vi "Craigslist Textbooks for Fusion Table V3.vi"() -> ()   [LabVIEW 2010]
uses:
  <vilib>/Utility/file.llb/Read From Spreadsheet File (string).vi
  <vilib>/Utility/file.llb/Write To Spreadsheet File (string).vi
panel:
  out "File Save Path":string
  out "Array":string[][](array[string])
  out "user books per city":string[][](array[string])
  out "Final filtered":string[][](array[string])
  out "element":string
  out "All closest city data":string[](array[string])
  out "All Data":string[][](array[string])
  out "ID number":string
  in  "Geo Locations 2":string[][](array[string])=[["http://boulder.craigslist.org/bks/", "http://boulder.craigslist.org/bks/index100.html", "http://boulder.craigslist.org/bks/index200.html", "http://boulder.craigslist.org/bks/index300.html", "http://boulder.craigslist.org/bks/index400.html", "http://boulder.craigslist.org/bks/index500.html", "http://boulder.craigslist.org/bks/index600.html", "http://boulder.craigslist.org/bks/index700.html", "http://boulder.craigslist.org/bks/index800.html", "http://boulder.craigslist.org/bks/index900.html", "40.006846", "-105.271575", "CU Boulder", "Boulder", "CO", "4/30/2004 7:48:47 PM", "3558694"], ["http://phoenix.craigslist.org/bks/", "http://phoenix.craigslist.org/bks/index100.html", "http://phoenix.craigslist.org/bks/index200.html", "http://phoenix.craigslist.org/bks/index300.html", "http://phoenix.craigslist.org/bks/index400.html", "http://phoenix.craigslist.org/bks/index500.html", "http://phoenix.craigslist.org/bks/index600.html", "http://phoenix.craigslist.org/bks/index700.html", "http://phoenix.craigslist.org/bks/index800.html", "http://phoenix.craigslist.org/bks/index900.html", "33.416147", "-111.938152", "ASU Arizona State University", "Phoenix", "AZ", "4/30/2004 7:48:47 PM", "3558688"], ["http://orlando.craigslist.org/bks/", "http://orlando.craigslist.org/bks/index100.html", "http://orlando.craigslist.org/bks/index200.html", "http://orlando.craigslist.org/bks/index300.html", "http://orlando.craigslist.org/bks/index400.html", "http://orlando.craigslist.org/bks/index500.html", "http://orlando.craigslist.org/bks/index600.html", "http://orlando.craigslist.org/bks/index700.html", "http://orlando.craigslist.org/bks/index800.html", "http://orlando.craigslist.org/bks/index900.html", "28.602326", "-81.19994", "UCF University of Central Florida", "orlando", "FL", "", "3558796"], ["http://austin.craigslist.org/bks/", "http://austin.craigslist.org/bks/index100.html", "http://austin.craigslist.org/bks/index200.html", "http://austin.craigslist.org/bks/index300.html", "http://austin.craigslist.org/bks/index400.html", "http://austin.craigslist.org/bks/index500.html", "http://austin.craigslist.org/bks/index600.html", "http://austin.craigslist.org/bks/index700.html", "http://austin.craigslist.org/bks/index800.html", "http://austin.craigslist.org/bks/index900.html", "30.28629", "-97.740211", "UT Austin University of Texas at Austin", "Austin", "TX", "40.006846", "3588692"], ["http://columbus.craigslist.org/bks/", "http://columbus.craigslist.org/bks/index100.html", "http://columbus.craigslist.org/bks/index200.html", "http:/columbus.craigslist.org/bks/index300.html", "http://columbus.craigslist.org/bks/index400.html", "http://columbus.craigslist.org/bks/index500.html", "http://columbus.craigslist.org/bks/index600.html", "http://columbus.craigslist.org/bks/index700.html", "http://columbus.craigslist.org/bks/index800.html", "http://columbus.craigslist.org/bks/index900.html", "40.000778", "-83.010421", "OSU Ohio State University", "Columbus", "OH", "4/30/2004 7:48:47 PM", "3558876"], ["http://minneapolis.craigslist.org/bks/", "http://minneapolis.craigslist.org/bks/index100.html", "http://minneapolis.craigslist.org/bks/index200.html", "http://minneapolis.craigslist.org/bks/index300.html", "http://minneapolis.craigslist.org/bks/index400.html", "http://minneapolis.craigslist.org/bks/index500.html", "http://minneapolis.craigslist.org/bks/index600.html", "http://minneapolis.craigslist.org/bks/index700.html", "http://minneapolis.craigslist.org/bks/index800.html", "http://minneapolis.craigslist.org/bks/index900.html", "44.974999", "-93.231847", "U of M University of Minnesota", "minneapolis", "MN", "", "3558694"], ["http://losangeles.craigslist.org/lac/bks/", "http://losangeles.craigslist.org/lac/bks/index100.html", "http://losangeles.craigslist.org/lac/bks/index200.html", "http://losangeles.craigslist.org/lac/bks/index300.html", "http://losangeles.craigslist.org/lac/bks/index400.html", "http://losangeles.craigslist.org/lac/bks/index500.html", "http://losangeles.craigslist.org/lac/bks/index600.html", "http://losangeles.craigslist.org/lac/bks/index700.html", "http://losangeles.craigslist.org/lac/bks/index800.html", "http://losangeles.craigslist.org/lac/bks/index900.html", "34.020612", "-118.284409", "USC University of Southern California", "USC", "CA", "40.006846", "3588399"], ["http://boston.craigslist.org/gbs/bks/", "http://boston.craigslist.org/gbs/bks/index100.html", "http://boston.craigslist.org/gbs/bks/index200.html", "http://boston.craigslist.org/gbs/bks/index300.html", "http://boston.craigslist.org/gbs/bks/index400.html", "http://boston.craigslist.org/gbs/bks/index500.html", "http://boston.craigslist.org/gbs/bks/index600.html", "http://boston.craigslist.org/gbs/bks/index700.html", "http://boston.craigslist.org/gbs/bks/index800.html", "http://boston.craigslist.org/gbs/bks/index900.html", "42.372852", "-71.117581", "Harvard University", "Cambridge", "MA", "40.006846", "3589108"], ["http://newhaven.craigslist.org/bks/", "http://newhaven.craigslist.org/bks/index100.html", "http://newhaven.craigslist.org/bks/index200.html", "http://newhaven.craigslist.org/bks/index300.html", "http://newhaven.craigslist.org/bks/index400.html", "http://newhaven.craigslist.org/bks/index500.html", "http://newhaven.craigslist.org/bks/index600.html", "http://newhaven.craigslist.org/bks/index700.html", "http://newhaven.craigslist.org/bks/index800.html", "http://newhaven.craigslist.org/bks/index900.html", "41.311211", "-72.928662", "Yale University", "New Haven", "CT", "40.006846", "3588844"], ["http://sfbay.craigslist.org/pen/bks/", "http://sfbay.craigslist.org/pen/bks/index100.html", "http://sfbay.craigslist.org/pen/bks/index200.html", "http://sfbay.craigslist.org/pen/bks/index300.html", "http://sfbay.craigslist.org/pen/bks/index400.html", "http://sfbay.craigslist.org/pen/bks/index500.html", "http://sfbay.craigslist.org/pen/bks/index600.html", "http://sfbay.craigslist.org/pen/bks/index700.html", "http://sfbay.craigslist.org/pen/index800.html", "http://sfbay.craigslist.org/pen/bks/index900.html", "37.425576", "-122.168891", "Stanford University", "Redwood City", "CA", "40.006846", "3588839"], ["http://chicago.craigslist.org/nch/bks/", "http://chicago.craigslist.org/nch/bks/index100.html", "http://chicago.craigslist.org/nch/bks/index200.html", "http://chicago.craigslist.org/nch/bks/index300.html", "http://chicago.craigslist.org/nch/bks/index400.html", "http://chicago.craigslist.org/nch/bks/index500.html", "http://chicago.craigslist.org/nch/bks/index600.html", "http://chicago.craigslist.org/nch/bks/index700.html", "http://chicago.craigslist.org/nch/bks/index800.html", "http://chicago.craigslist.org/nch/bks/index900.html", "42.057801", "-87.67563", "NU Northwestern University", "Evanston", "IL", "40.006846", "3588099"], ["http://sfbay.craigslist.org/eby/bks/", "http://sfbay.craigslist.org/eby/bks/index100.html", "http://sfbay.craigslist.org/eby/bks/index200.html", "http://sfbay.craigslist.org/eby/bks/index300.html", "http://sfbay.craigslist.org/eby/bks/index400.html", "http://sfbay.craigslist.org/eby/bks/index500.html", "http://sfbay.craigslist.org/eby/bks/index600.html", "http://sfbay.craigslist.org/eby/bks/index700.html", "http://sfbay.craigslist.org/eby/bks/index800.html", "http://sfbay.craigslist.org/eby/bks/index900.html", "37.872296", "-122.258799", "UC Berkeley University of California at Berkeley", "Berkeley", "CA", "40.006846", "3588671"], ["http://fortcollins.craigslist.org/bks/", "http://fortcollins.craigslist.org/bks/index100.html", "http://fortcollins.craigslist.org/bks/index200.html", "http://fortcollins.craigslist.org/bks/index300.html", "http://fortcollins.craigslist.org/bks/index400.html", "http://fortcollins.craigslist.org/bks/index500.html", "http://fortcollins.craigslist.org/bks/index600.html", "http://fortcollins.craigslist.org/bks/index700.html", "http://fortcollins.craigslist.org/bks/index800.html", "http://fortcollins.craigslist.org/bks/index900.html", "40.571556", "-105.080624", "CSU Colorado State University", "Fort Collins", "CO", "40.006846", "3589102"], ["http://denver.craigslist.org/bks/", "http://denver.craigslist.org/bks/index100.html", "http://denver.craigslist.org/bks/index200.html", "http://denver.craigslist.org/bks/index300.html", "http://denver.craigslist.org/bks/index400.html", "http://denver.craigslist.org/bks/index500.html", "http://denver.craigslist.org/bks/index600.html", "http://denver.craigslist.org/bks/index700.html", "http://denver.craigslist.org/bks/index800.html", "http://denver.craigslist.org/bks/index900.html", "39.676707", "-104.962628", "DU University of Denver", "Denver", "CO", "40.006846", "3588279"], ["http://boston.craigslist.org/gbs/bks/", "http://boston.craigslist.org/gbs/bks/index100.html", "http://boston.craigslist.org/gbs/bks/index200.html", "http://boston.craigslist.org/gbs/bks/index300.html", "http://boston.craigslist.org/gbs/bks/index400.html", "http://boston.craigslist.org/gbs/bks/index500.html", "http://boston.craigslist.org/gbs/bks/index600.html", "http://boston.craigslist.org/gbs/bks/index700.html", "http://boston.craigslist.org/gbs/bks/index800.html", "http://boston.craigslist.org/gbs/bks/index900.html", "42.361556", "-71.090759", "MIT Massachusetts Institute of Technology", "Cambridge", "MA", "40.006846", "3588278"]]
  out "Finished Array":string[][](array[string])
  out "One Row Edited":string[](array[string])
  out "Craigslist Link":string
  out "Place":string
  out "One Row Unedited":string[](array[string])
  out "Category":string
  out "Extra Information":string
  out "Price":string
  out "General Location":string
  out "Time":string
  out "Date":string
  out "Year":string
  out "Date, Time":string
  out "State":string
  out "City":string
  out "long string":string
  out "lat string":string
  out "Full Source":string
  out "long":dbl
  out "lat":dbl
  out "Body":string
  out "E-mail Contact":string
  out "Title":string
  out "Parse Count":i32
  out "Current Page Source":string
  # "http://thestudentbookproject.org/index2.php?option=com_google_maps_boulder&task=dynamic&no_html=1&download=true&zip=false"
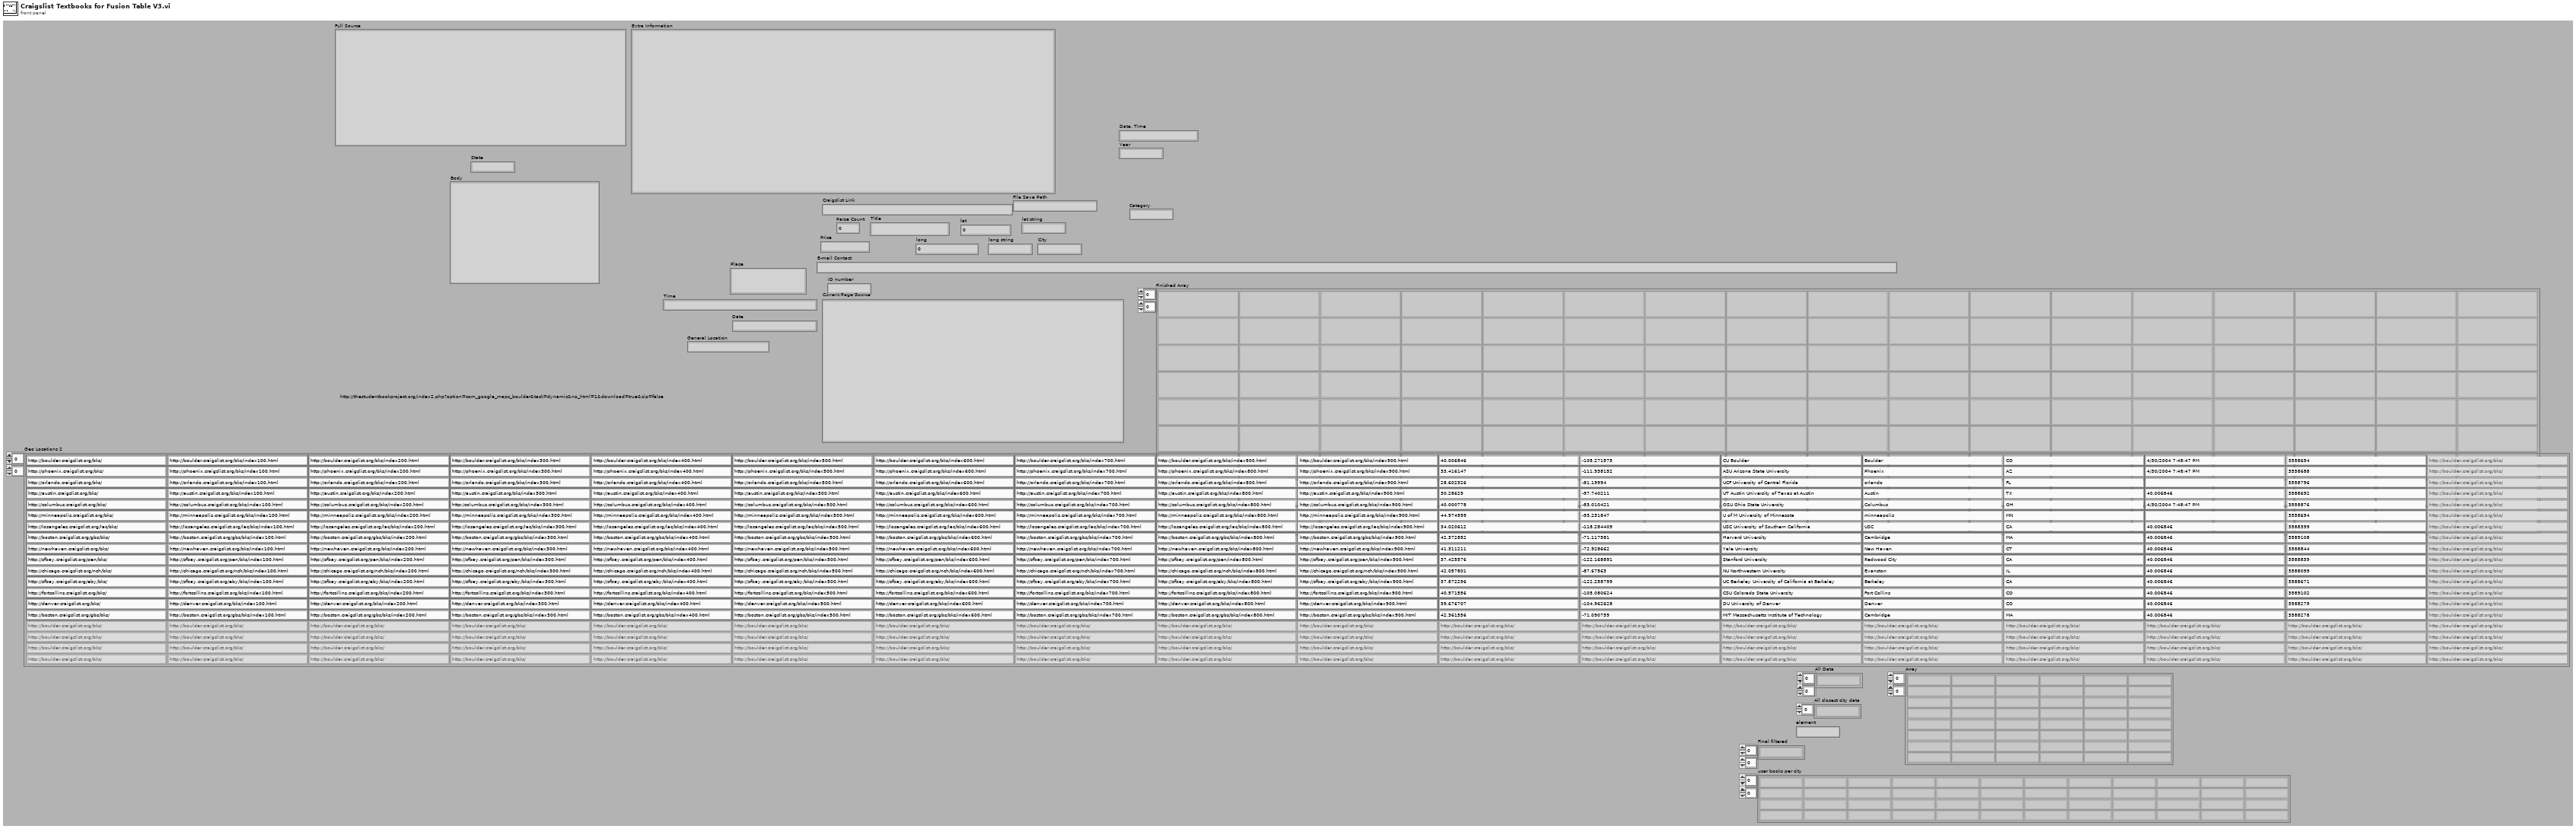
[diagram p1: front panel]
types:
  T1 = enum16{"open", "replace", "create", "open or create", "replace or create", "replace or create with confirmation"}
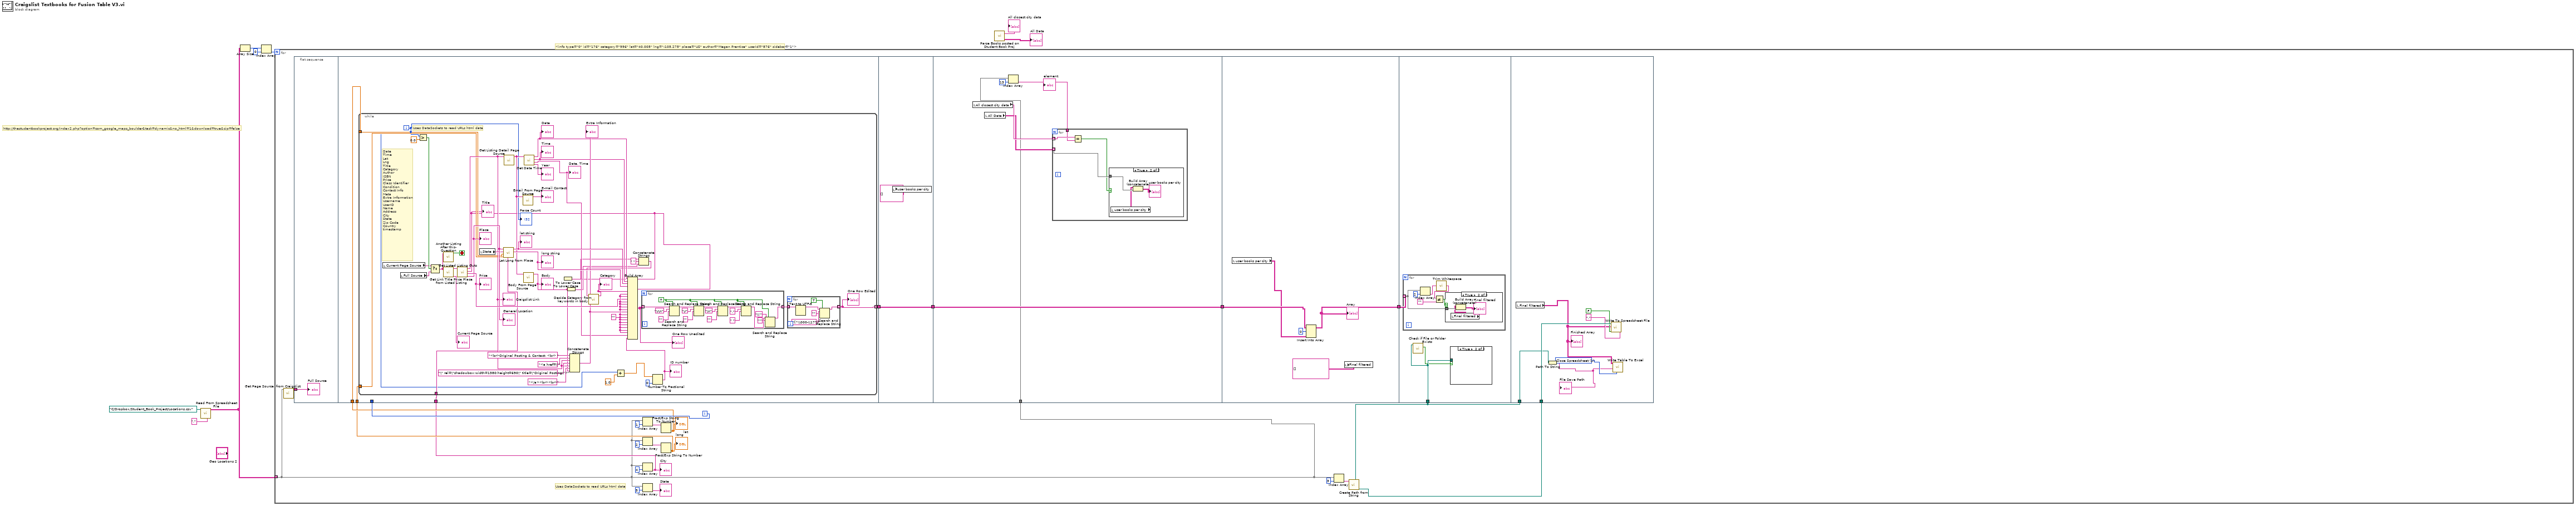
[diagram p0: block diagram]
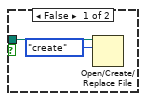
[diagram p3: hidden frame]
diagram:
  # "http://thestudentbookproject.org/index2.php?option=com_google_maps_boulder&task=dynamic&no_html=1&download=true&zip=false"
  # "<info type=\"0\" id=\"176\" category=\"996\" lat=\"40.005\" lng=\"-105.275\" place=\"US\" author=\"Megan Prentice\" userid=\"876\" sidebar=\"1\">"
  n1 = call-poly <vilib>:"Read From Spreadsheet File.vi"("delimiter (\\t)"="," ("delimiter (\\t)"), "file path (dialog if empty)"=path "C:/Dropbox/Student_Book_Project/Locations.csv") -> ("all rows"=w3:string[][])  [unwired: 5 in, 4 out]
  n2 = Array Size(array=w3) -> (size(s)=w8:i32[])
  n3 = Index Array(array=w8, index=0) -> (element=w6:i32)
  n4 = for {
    N: w6 -> [_]
    tunnel: w3 -> [w12] mode=indexing
    i -> [w21]
    # "Uses DataSockets to read URLs html data"
    n5 = call "Get Page Source  from Craigslist.vi"("Input Vaiables Array"=w12) -> ("Full Page Source of 9 pages combined"=w19:string)  [unwired: 10 in]
    n6 = flat-sequence {
      tunnel: w19 -> [w30]
      tunnel: w21 -> [_]
      tunnel: [w34] -> w11
      tunnel: w18 -> [w33]
      tunnel: w17 -> [w32]
      tunnel: w16 -> [w31]
      tunnel: w11 -> [w103]
      tunnel: [w103] -> w10
      tunnel: [w109] -> w13
      tunnel: w12 -> [w104]
      tunnel: w10 -> [w109]
      tunnel: w13 -> [w120]
      tunnel: [w117] -> w14
      tunnel: w14 -> [w124]
      tunnel: w9 -> [w123]
      tunnel: w9 -> [w139]
      tunnel: w20 -> [w142]
      frame #0 {
        "Full Source" <- w30
      }
      frame #1 {
        n7 = while {
          tunnel: [w50] -> w34 mode=indexing
          tunnel: w33 -> [w54]
          tunnel: w32 -> [w53]
          tunnel: w31 -> [w42]
          i -> [w39]
          stop <- w69 stop-if-true
          w70 = "" ("element")
          # "Date\nTime\nLat\nLng\nTitle\nCategory\nAuthor\nISBN\nPrice\nClass Identifier\nCondition\nContact Info\nMeta\nExtra Information\nUsername\nUserID\nName\nAddress\nCity\nState\nZip Code \nCountry\ntimestamp"
          # "Uses DataSockets to read URLs html data"
          n8 = local read "Current Page Source"() -> (w76:string)
          n9 = local read "Full Source"() -> (w75:string)
          n10 = Greater?(x=w39, y=0.0) -> (0:w77:bool)
          n11 = Select(t=w76, s=w77, f=w75) -> (s? t:f=w68:string)
          n12 = call "Another Listing After this- Question.vi"("Current Page Source"=w68) -> ("Another Listing After"=w69:bool)  [unwired: 10 in]
          n13 = call "Get Listed Listing Guts.vi"("Current Page Source"=w68) -> ("Updated Page Source"=→"Current Page Source":string, "Listed Listing Guts"=w66:string)  [unwired: 9 in]
          n14 = call "Get Link Title Price Place from Listed Listing.vi"("Listed Listing Guts"=w66) -> ("Place"=w64:string, "Price w/ $ sign"=w65:string, "Listing Title"=w35:string, "Craigslist Link"=w60:string)  [unwired: 7 in]
          "Title" <- w35
          "General Location" <- w64
          "Price" <- w65
          "Place" <- w64
          "Craigslist Link" <- w60
          n15 = local read "State"() -> (w63:string)
          n16 = call "Lat Long from Place.vi"("City default name"=w42, "Long"=w53, "Lat"=w54, "County/State"=w63, "CL Place Name"=w64) -> ("long string"=w61:string, "lat string"=w62:string)  [unwired: 5 in]
          "lat string" <- w62
          "long string" <- w61
          n17 = call "Get Listing Detail Page Source.vi"("URL"=w60) -> ("Page Source"=w58:string)  [unwired: 10 in]
          n18 = call "Email From Page Source.vi"("Detail Page Source"=w58) -> ("E-mail Contact"=→"E-mail Contact":string)  [unwired: 10 in]
          n19 = call "Body From Page Source.vi"("Detail Page Source"=w58) -> ("Body (Body, Images, Location, Everything)"=w56:string)  [unwired: 10 in]
          "Body" <- w56
          n20 = call "Get Date Time.vi"("Detail Page Source"=w58) -> ("Year"=→"Year":string, "Date, Time"=w47:string, "Time"=w48:string, "Date"=w49:string)  [unwired: 7 in]
          "Date, Time" <- w47
          "Date" <- w49
          "Time" <- w48
          n21 = To Lower Case(string=w35) -> (all lower case string=w46:string)
          n22 = To Lower Case(string=w56) -> (all lower case string=w45:string)
          n23 = Concatenate Strings("<br>Original Posting & Contact: <br> " ("string"), "<a href=\"" ("string"), w60, "\" rel=\"shadowbox;width=1380;height=690\" title=\"Original Posting\">" ("string"), w60, "</a><br><br>" ("string"), w56) -> (w55:string)
          "Extra Information" <- w55
          n24 = Add(x=w39, y=1.0) -> (x+y=w38:dbl)
          n25 = Concatenate Strings(w46, " " ("string"), w45) -> (w44:string)
          n26 = call "Decide Category from keywords in body.vi"("Body of Posting to Search"=w44) -> ("Category Determined"=w37:string)  [unwired: 10 in]
          "Category" <- w37
          n27 = Number To Fractional String(number=w38, precision (6)=i16 0) -> (F-format string=w40:string)  [unwired: 2 in]
          "ID number" <- w40
          n28 = Build Array(w49, w48, w62, w61, w35, w37, w70, w70, w65, w70, w70, w70, w70, w55, w70, w70, w70, w70, w70, w70, w70, w70, w47, w40) -> (w52:string[])
          "One Row Unedited" <- w52
          n29 = for {
            tunnel: w52 -> [w101] mode=indexing
            tunnel: [w86] -> w51 mode=indexing
            w85 = TRUE ("replace all? (F)")
            n30 = Search and Replace String(replace all?=w85, input string=w101, search string="\r\n", replace string="" ("replace string (\"\")")) -> (result string=w96:string)  [unwired: 4 in, 3 out]
            n31 = Search and Replace String(replace all?=w85, input string=w96, search string="\r", replace string="" ("replace string (\"\")")) -> (result string=w95:string)  [unwired: 4 in, 3 out]
            n32 = Search and Replace String(replace all?=w85, input string=w95, search string="\n", replace string="" ("replace string (\"\")")) -> (result string=w90:string)  [unwired: 4 in, 3 out]
            n33 = Search and Replace String(replace all?=w85, input string=w90, search string=",", replace string=" " ("replace string (\"\")")) -> (result string=w87:string)  [unwired: 4 in, 3 out]
            n34 = Search and Replace String(replace all?=w85, input string=w87, search string="'", replace string="\\'" ("replace string (\"\")")) -> (result string=w86:string)  [unwired: 4 in, 3 out]
          }
          n35 = for {
            tunnel: w51 -> [w84] mode=indexing
            tunnel: [w81] -> w50 mode=indexing
            n36 = Text to UTF-8(11:w84) -> (3:w82:string)  [unwired: 1 in, 1 out]
            n37 = Search and Replace String(replace all?=TRUE ("replace all? (F)"), input string=w82, search string="[^\\000-\\177]", replace string="" ("replace string (\"\")")) -> (result string=w81:string)  [unwired: 4 in, 3 out]
          }
          "One Row Edited" <- w50
          "Parse Count" <- w39
        }
      }
      frame #2 {
        n38 = local write "user books per city"(string[][] [] ("user books per city")) -> ()
      }
      frame #3 {
        n39 = local read "All closest city data"() -> (w107:string[])
        n40 = local read "All Data"() -> (w105:string[][])
        n41 = Index Array(array=w104, index=13) -> (element=w106:string)
        "element" <- w106
        n42 = for {
          tunnel: w107 -> [w113] mode=indexing
          tunnel: w106 -> [w112]
          tunnel: w105 -> [w111] mode=indexing
          n43 = Equal?(x=w113, y=w112) -> (x = y?=w110:bool)
          n44 = case shown="True" w110 {
            tunnel: w111 -> [_ w116]
            frame False {
            }
            frame True {
              n45 = local read "user books per city"() -> (w114:string[][])
              n46 = Build Array (concatenate)(w114, w116) -> (→"user books per city":string[][])
            }
          }
        }
      }
      frame #4 {
        n47 = local read "user books per city"() -> (w118:string[][])
        n48 = Insert Into Array(array=w120, index (row)=0, new element=w118) -> (w117:string[][])  [unwired: 1 in]
        "Array" <- w117
        n49 = local write "Final filtered"(string[][] [] ("Final filtered")) -> ()
      }
      frame #5 {
        n50 = for {
          tunnel: w124 -> [w130] mode=indexing
          n51 = Index Array(array=w130, index=2) -> (element=w129:string)
          n52 = call <vilib>:"Trim Whitespace.vi"("string"=w129) -> ("trimmed string"=w128:string)  [unwired: 1 in]
          n53 = Not Equal?(x=w128, y="") -> (x != y?=w131:bool)
          n54 = case shown="True" w131 {
            tunnel: w130 -> [_ w135]
            frame False {
            }
            frame True {
              n55 = local read "Final filtered"() -> (w133:string[][])
              n56 = Build Array (concatenate)(w133, w135) -> (→"Final filtered":string[][])
            }
          }
        }
        n57 = call <vilib>:"Check if File or Folder Exists.vi"("path"=w123) -> ("file or folder exists?"=w122:bool)  [unwired: 8 in, 2 out]
        n58 = case shown="True" w122 {
          tunnel: w123 -> [w125 _]
          frame False {
            n59 = Open/Create/Replace File(file path (use dialog)=w125, operation (0:open)=T1."create") -> ()  [unwired: 4 in, 3 out]
          }
          frame True {
          }
        }
      }
      frame #6 {
        w137 = u16 1 items=["Leave Excel Open", "Close Spreadsheet"] ("Completion Task")
        n60 = local read "Final filtered"() -> (w138:string[][])
        "Finished Array" <- w138
        n61 = Path To String(path=w139) -> (string=w136:string)
        "File Save Path" <- w136
        n62 = call-poly <vilib>:"Write To Spreadsheet File.vi"("delimiter (\\t)"="," ("delimiter (\\t)"), "append to file? (new file:F)"=FALSE, "2D data"=w138, "file path (dialog if empty)"=w142) -> ()  [unwired: 4 in, 1 out]
        n63 = call "Write Table To Excel.vi"("Table"=w138, "Filename"=w136, "Completion Task"=w137) -> ()  [unwired: 4 in]
      }
    }
    n64 = Index Array(array=w12, index=1) -> (element=w27:string)
    n65 = Index Array(array=w12, index=2) -> (element=w26:string)
    n66 = Index Array(array=w12, index=4) -> (element=w16:string)
    "City" <- w16
    n67 = Index Array(array=w12, index=5) -> (element=→"State":string)
    n68 = Fract/Exp String To Number(string=w27) -> (number=w18:dbl)  [unwired: 3 in, 1 out]
    "lat" <- w18
    n69 = Fract/Exp String To Number(string=w26) -> (number=w17:dbl)  [unwired: 3 in, 1 out]
    "long" <- w17
    n70 = Index Array(array=w12, index=3) -> (element=w15:string)
    n71 = call "Create Path from String.vi"("Folder Name (CU Boulder)"=w15) -> ("Permanent Path"=w20:path, "Google Docs Path"=w9:path)  [unwired: 9 in]
  }
  n72 = call "Parse Books posted on Student Book Proj.vi"() -> ("All Data"=→"All Data":string[][], "All closest city data"=→"All closest city data":string[])  [unwired: 2 in]
